vi "Loop_ACT_Elbow.vi"() -> ()   [LabVIEW 2017, in "Arm.lvlib"]
uses:
  Arm.lvlib
  CLUSTER_ElbowOutput.ctl
  CLUSTER_ElbowInput.ctl
  Public/Documents/Cross The Road Electronics/Phoenix-LabVIEW/Motor Controller/Controls/CTRE_Phoenix_MotorControl_ControlMode.ctl
  TypeDef/CLUSTER_PID.ctl
  CONTROL_PositonGraph.ctl
  Public/Documents/Cross The Road Electronics/Phoenix-LabVIEW/Motor Controller/Controls/CTRE_Phoenix_MotorControl_FeedbackDevice.ctl
  Globals/Global_STOP.vi
  Global_SM Write_Data Out.vi
  Public/Documents/Cross The Road Electronics/Phoenix-LabVIEW/Motor Controller/Get/CTRE_Phoenix_MotorController_GetSelectedSensorData.vi
  Public/Documents/Cross The Road Electronics/Phoenix-LabVIEW/Motor Controller/Get/CTRE_Phoenix_MotorController_GetVoltage.vi
  Global_ACT Write_Data Out.vi
  <vilib>/Rock Robotics/WPI/RobotDrive/WPI_RobotDriveOpen2MotorWithExistingMotors.vi
  Globals/Global_Device_IDs.vi
panel:
  in  "Display Graph":bool
  out "Position Closed Loop Plots":T1
  out "Elbow Input":T2 {"Talon Mode" items=["PercentOutput"=0, "Position"=1, "Velocity"=2, "Current"=3, "Follower"=5, "MotionProfile"=6, "MotionMagic"=7, "MotionMagicArc"=8, "MotionProfileArc"=10, "Disabled"=15]}
  out "Elbow Output":T5
  out "Cycle Time (S)":dbl format="%.3g"
  in  "Target Time(ms)":u32=50
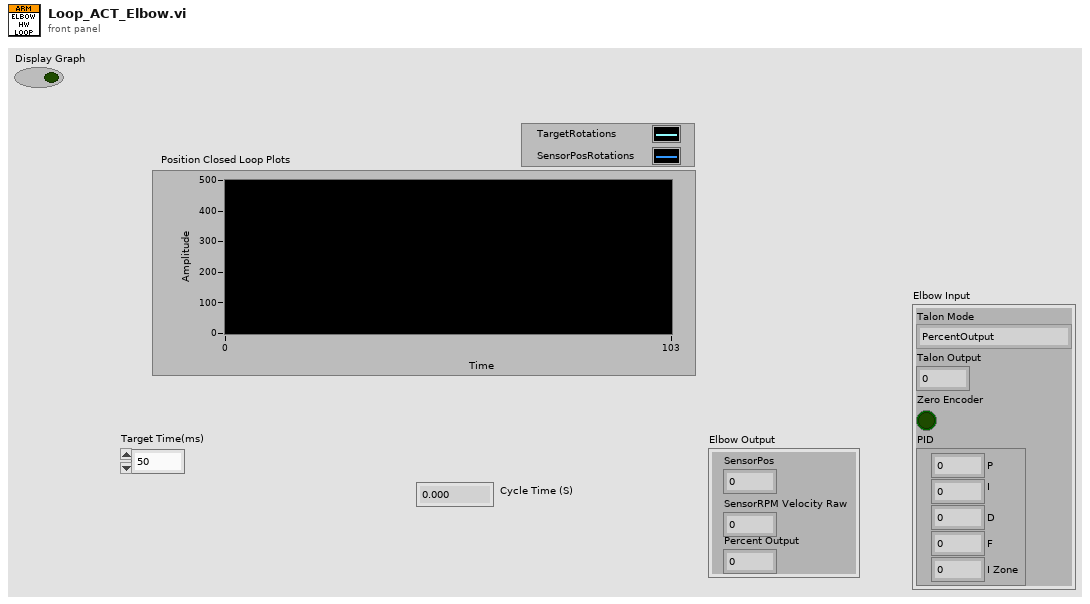
[diagram p1: front panel]
types:
  T1 = typedef "Arm.lvlib/CONTROL_PositonGraph.ctl" = cluster{dbl, "Position (Raw Sensor Units)":i32}
  T2 = typedef "Arm.lvlib/CLUSTER_ElbowInput.ctl" = cluster{"Talon Mode":T3, "Talon Output":dbl, "Zero Encoder":bool, "PID":T4}
  T3 = typedef "CTRE_Phoenix_MotorControl_ControlMode.ctl" = u16
  T4 = typedef "CLUSTER_PID.ctl" = cluster{"P":dbl, "I":dbl, "D":dbl, "F":dbl, "I Zone":dbl}
  T5 = typedef "Arm.lvlib/CLUSTER_ElbowOutput.ctl" = cluster{"SensorPos":i32, "SensorRPM Velocity Raw":i32, "Percent Output":dbl}
  T6 = typedef "CTRE_Phoenix_MotorControl_FeedbackDevice.ctl" = i8
  T7 = typedef "CLUSTER_Arm_Device_IDs.ctl" = cluster{"Elbow Setup":T8, "Telescope Setup":T8, "Wrist Setup":T8}
  T8 = typedef "CLUSTER_Talon_Setup.ctl" = cluster{"Talon SRX ID":u8, "PhaseSensor":bool, "Invert Motor?":bool, "Phoenix Feedback Select":T6, "pidLoopldx":i32, "PID":T4}
  T9 = typedef "WPI_MotorControlDeviceRef.ctl" = cluster{"DeviceStatus":errorcluster, "Type":T10, "PWM":cluster{"PWM Channel":T11, "DeadBand":T12}, "CAN":cluster{"Device Number":u8, "SetOutput VI Ref":variant, "GetOutput VI Ref":variant, "Enable VI Ref":variant, "Disable VI Ref":variant, "Data":variant}, "Invert":bool, "DIO PWM":cluster{"PWM \"Enable\" Channel":T11, "DIOChannel":T13, "PWM Rate":dbl}}
  T10 = typedef "WPI_MotorControlType.ctl" = enum16{"PWM", "CAN", "DIO PWM"}
  T11 = typedef "FPGA_DIOPWMChannel.ctl" = enum8{"PWM 0", "PWM 1", "PWM 2", "PWM 3", "PWM 4", "PWM 5", "PWM 6", "PWM 7", "PWM 8", "PWM 9", "PWM MXP 0", "PWM MXP 1", "PWM MXP 2", "PWM MXP 3", "PWM MXP 4", "PWM MXP 5", "PWM MXP 6", "PWM MXP 7", "PWM MXP 8", "PWM MXP 9", "Invalid"}
  T12 = typedef "WPI_PWMDeadband.ctl" = cluster{"Name":string, "maxPositivePwm":i32, "minPositivePwm":i32, "centerPwm":i32, "maxNegativePwm":i32, "minNegativePwm":i32, "angularRange":u16}
  T13 = typedef "FPGA_DIOChannel.ctl" = enum8{"DIO 0", "DIO 1", "DIO 2", "DIO 3", "DIO 4", "DIO 5", "DIO 6", "DIO 7", "DIO 8", "DIO 9", "DIO MXP 0", "DIO MXP 1", "DIO MXP 2", "DIO MXP 3", "DIO MXP 4", "DIO MXP 5", "DIO MXP 6", "DIO MXP 7", "DIO MXP 8", "DIO MXP 9", "DIO MXP 10", "DIO MXP 11", "DIO MXP 12", "DIO MXP 13", "DIO MXP 14", "DIO MXP 15", "SPI Port CS1", "SPI Port CS2", "SPI Port CS3", "SPI Port MISO", "SPI Port MOSI", "Invalid"}
  T14 = cluster{"PhoenixMotorControlDevRef":T9, "Elbow Output":T5, "Elbow Input":T2, "Target Time(ms)":u32, "Current Time":timestamp, "Previous Time":timestamp, "Cycle Time (S)":dbl, "Last PID":T4}
  T15 = typedef "WPI_RobotDriveDevRef.ctl" = cluster{"DevStatus":errorcluster, "Motors[]":T9[], "Square Inputs":bool, "Max Output":dbl}
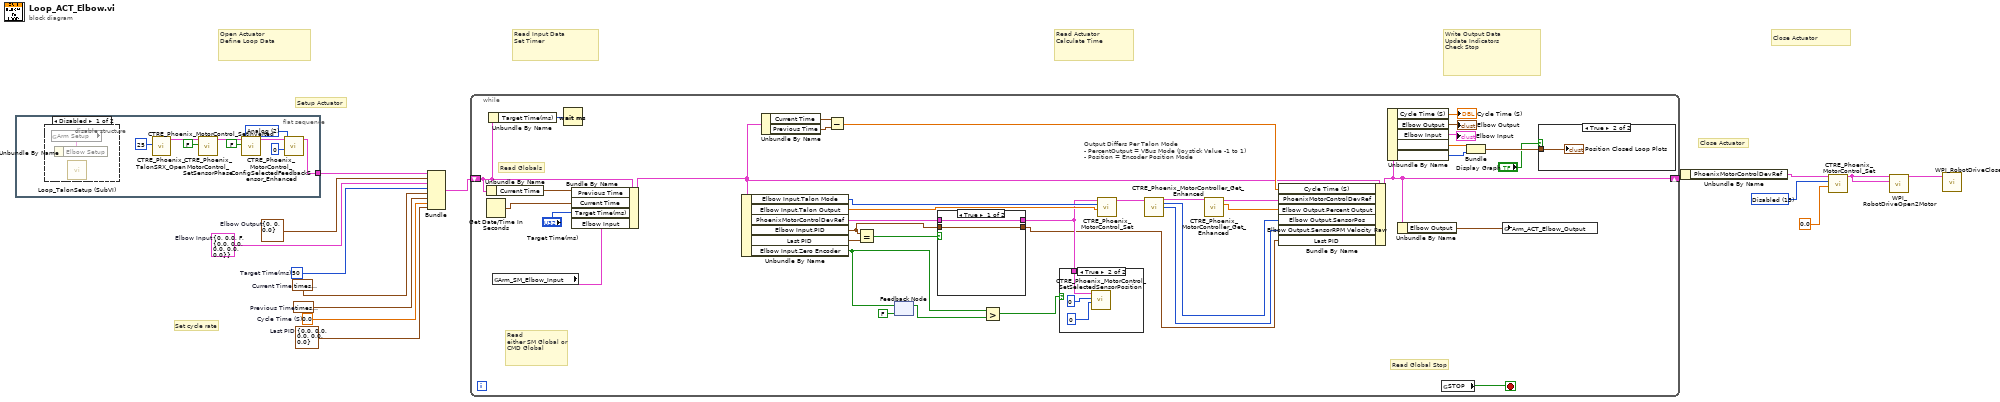
[diagram p0: block diagram]
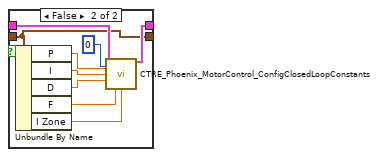
[diagram p3: hidden frame]
diagram:
  w2 = T4 {"P"=0.0, "I"=0.0, "D"=0.0, "F"=0.0, "I Zone"=0.0}  # Last PID
  w6 = T3 15 items=["PercentOutput"=0, "Position"=1, "Velocity"=2, "Current"=3, "Follower"=5, "MotionProfile"=6, "MotionMagic"=7, "MotionMagicArc"=8, "MotionProfileArc"=10, "Disabled"=15] ("Control Mode")
  w8 = T5 {"SensorPos"=0, "SensorRPM Velocity Raw"=0, "Percent Output"=0.0}  # Elbow Output
  w9 = T2 {"Talon Mode"=0, "Talon Output"=0.0, "Zero Encoder"=FALSE, "PID"={"P"=0.0, "I"=0.0, "D"=0.0, "F"=0.0, "I Zone"=0.0}}  # Elbow Input
  w10 = 0.0  # Cycle Time (S)
  w15 = timestamp(0 s since 1904-01-01)  # Previous Time
  w14 = timestamp(0 s since 1904-01-01)  # Current Time
  w13 = u32 50  # Target Time(ms)
  # "Close Actuator"
  # "Write Output Data\nUpdate Indicators\nCheck Stop"
  # "Read Actuator\nCalculate Time"
  # "Read Input Data\nSet Timer"
  # "Open Actuator\nDefine Loop Data"
  # "Set cycle rate"
  # "Close Actuator"
  # "Setup Actuator"
  n1 = flat-sequence {
    tunnel: [w21] -> w1
    frame #0 {
      w20 = T6 2 items=["None"=-1, "QuadEncoder"=0, "Analog"=2, "Tachometer"=4, "Pulse Width Encoded Position"=8, "Sensor Sum (S0 + S1)"=9, "Sensor Difference (D0 - D1)"=10, "Remote Source 0"=11, "Remote Source 1"=12, "Software Emulated"=15] ("Feedback Device")
      n2 = disable-structure shown="Disabled" {
        frame Disabled {
          n3 = global read "Global_Device_IDs.vi" "Arm Setup"() -> (w25:T7)
          n4 = Unbundle By Name(w25) -> ()  [unwired: 1 out]
          n5 = call "Loop_TalonSetup (SubVI).vi"() -> ()  [unwired: 11 in, 1 out]
        }
        frame Enabled {
        }
      }
      n6 = call "CTRE_Phoenix_TalonSRX_Open.vi"("Device Number"=u8 25) -> ("CAN Talon SRX Ref"=w24:T9)  [unwired: 9 in, 1 out]
      n7 = call "CTRE_Phoenix_MotorControl_SetSensorPhase.vi"("PhaseSensor"=FALSE, "PhoenixMotorControlDevRef"=w24) -> ("PhoenixMotorControlDevRef"=w23:T9)  [unwired: 8 in, 1 out]
      n8 = call "CTRE_Phoenix_MotorControl_SetInverted.vi"("Invert?"=FALSE, "PhoenixMotorControlDevRef"=w23) -> ("PhoenixMotorControlDevRef"=w22:T9)  [unwired: 8 in, 1 out]
      n9 = call "CTRE_Phoenix_MotorControl_ConfigSelectedFeedbackSensor_Enhanced.vi"("pidLoopIdx"=0, "Feedback Device"=w20, "PhoenixMotorControlDevRef"=w22) -> ("PhoenixMotorControlDevRef"=w21:T9)  [unwired: 7 in, 1 out]
    }
  }
  n10 = Bundle("PhoenixMotorControlDevRef"=w1, "Elbow Output"=w8, "Elbow Input"=w9, "Target Time(ms)"=w13, "Current Time"=w14, "Previous Time"=w15, "Cycle Time (S)"=w10, "Last PID"=w2) -> (w12:T14)  [unwired: 1 in]
  n11 = while {
    shift-right: [w55] -> w11
    shift-left: w12 -> [w57]
    stop <- w63 stop-if-true
    # "Output Differs Per Talon Mode\n- PercentOutput = VBus Mode (Joystick Value -1 to 1)\n- Position = Encoder Position Mode"
    # "Read\neither SM Global or CMD Global"
    # "Read Globals"
    # "Read Global Stop"
    n12 = Unbundle By Name(w57) -> ("Current Time"=w61:timestamp)
    n13 = Get Date/Time In Seconds() -> (seconds since 1Jan1904=w62:timestamp)
    n14 = Unbundle By Name(w57) -> ("Target Time(ms)"=w56:u32)
    n15 = global read "Global_SM Write_Data Out.vi" "Arm_SM_Elbow_Input"() -> (w51:T2)
    n16 = Wait (ms)(milliseconds to wait=w56) -> ()  [unwired: 1 out]
    n17 = Bundle By Name(cluster=w57, "Previous Time"=w61, "Current Time"=w62, "Target Time(ms)"="Target Time(ms)", "Elbow Input"=w51) -> (w38:T14)
    n18 = Unbundle By Name(w38) -> ("Elbow Input.Talon Mode"=w50:T3, "Elbow Input.Talon Output"=w49:dbl, "PhoenixMotorControlDevRef"=w37:T9, "Elbow Input.PID"=w33:T4, "Last PID"=w34:T4, "Elbow Input.Zero Encoder"=w28:bool)
    n19 = Unbundle By Name(w38) -> ("Current Time"=w60:timestamp, "Previous Time"=w59:timestamp)
    n20 = Subtract(x=w60, y=w59) -> (x-y=w53:dbl)
    n21 = Equal?(x=w33, y=w34) -> (x = y?=w31:bool)
    n22 = feedback #1(FALSE) -> (w29:bool)
    n23 = feedback-in #1(w28) -> ()
    n24 = case shown="True" w31 {
      tunnel: w37 -> [w65 w74]
      tunnel: [w65 w73] -> w36
      tunnel: w33 -> [w64 w66]
      tunnel: [w64 w66] -> w32
      frame True {
      }
      frame False {
        n25 = Unbundle By Name(w66) -> ("P"=w71:dbl, "I"=w70:dbl, "D"=w69:dbl, "F"=w68:dbl, "I Zone"=w67:dbl)
        n26 = call "CTRE_Phoenix_MotorControl_ConfigClosedLoopConstants.vi"("PhoenixMotorControlDevRef"=w74, "slotIdx"=0, "P"=w71, "I"=w70, "D"=w69, "F"=w68, "I Zone"=w67) -> ("PhoenixMotorControlDevRef"=w73:T9)  [unwired: 7 in, 1 out]
      }
    }
    n27 = Greater?(x=w28, y=w29) -> (0:w27:bool)
    n28 = case shown="True" w27 {
      tunnel: w36 -> [_ w78]
      frame False {
      }
      frame True {
        n29 = call "CTRE_Phoenix_MotorControl_SetSelectedSensorPosition.vi"("pidLoopIdx"=u32 0, "New Sensor Position"=0, "PhoenixMotorControlDevRef"=w78) -> ()  [unwired: 7 in, 2 out]
      }
    }
    n30 = call "CTRE_Phoenix_MotorControl_Set.vi"("Output"=w49, "Control Mode"=w50, "PhoenixMotorControlDevRef"=w36) -> ("PhoenixMotorControlDevRef"=w48:T9)  [unwired: 7 in, 1 out]
    n31 = call-poly "CTRE_Phoenix_MotorController_Get_Enhanced.vi"("PhoenixMotorControlDevRef"=w48) -> ("PhoenixMotorControlDevRef"=w47:T9, "Position (Raw Sensor Units)"=w44:i32, "Velocity (Raw Sensor Units per 100 ms)"=w45:i32)  [unwired: 11 in, 1 out]
    n32 = call-poly "CTRE_Phoenix_MotorController_Get_Enhanced.vi"("PhoenixMotorControlDevRef"=w47) -> ("PhoenixMotorControlDevRef"=w26:T9, "Percent Output"=w46:dbl)  [unwired: 10 in, 3 out]
    n33 = Bundle By Name(cluster=w38, "Cycle Time (S)"=w53, "PhoenixMotorControlDevRef"=w26, "Elbow Output.Percent Output"=w46, "Elbow Output.SensorPos"=w44, "Elbow Output.SensorRPM Velocity Raw"=w45, "Last PID"=w32) -> (w55:T14)
    n34 = Unbundle By Name(w55) -> ("Cycle Time (S)"=→"Cycle Time (S)":dbl, "Elbow Output"=→"Elbow Output":T5, "Elbow Input"=→"Elbow Input":T2, "Elbow Input.Talon Output"=w41:dbl, "Elbow Output.SensorPos"=w40:i32)
    n35 = Unbundle By Name(w55) -> ("Elbow Output"=w52:T5)
    n36 = global read "Global_STOP.vi" "STOP"() -> (w63:bool)
    n37 = Bundle("Talon Output"=w41, "SensorPos"=w40) -> (w39:cluster{"Talon Output":dbl, "SensorPos":i32})  [unwired: 1 in]
    n38 = global write "Global_ACT Write_Data Out.vi" "Arm_ACT_Elbow_Output"(w52) -> ()
    n39 = case shown="True" "Display Graph" {
      tunnel: w39 -> [_ w75]
      frame False {
      }
      frame True {
        "Position Closed Loop Plots" <- w75
      }
    }
  }
  n40 = Unbundle By Name(w11) -> ("PhoenixMotorControlDevRef"=w7:T9)
  n41 = call "CTRE_Phoenix_MotorControl_Set.vi"("Output"=0.0, "Control Mode"=w6, "PhoenixMotorControlDevRef"=w7) -> ("PhoenixMotorControlDevRef"=w3:T9)  [unwired: 7 in, 1 out]
  n42 = call-poly <vilib>:"WPI_RobotDriveOpen2Motor.vi"("Right Motor Dev Ref"=w3, "Left Motor Dev Ref"=w3) -> ("RobotDriveDevRef"=w5:T15)  [unwired: 8 in, 1 out]
  n43 = call <vilib>:"WPI_RobotDriveClose.vi"("RobotDriveDevRef"=w5) -> ()  [unwired: 10 in, 1 out]
